vi "CheckPYME.vi"(0 "Anos de tu negocio":i32, 5 "Garantia":dbl, 7 "Importe total":dbl, 9 "Flujo de efectivo mensual":dbl, 11 "Numero de sucursales":i32) -> (6 "Sujeto a credito?":bool, 8 "Puntos momentaneos":i32, 10 "Status":string)   [LabVIEW 2018]
doc: "Verifica si la PYME esta sujeta a credito o no"
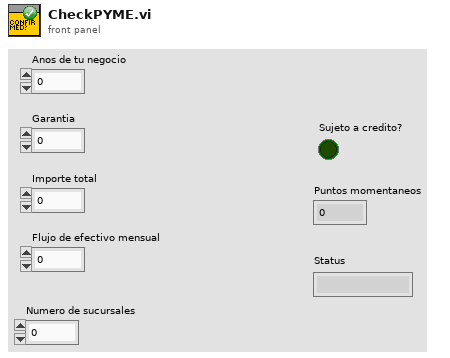
[diagram p1: front panel]
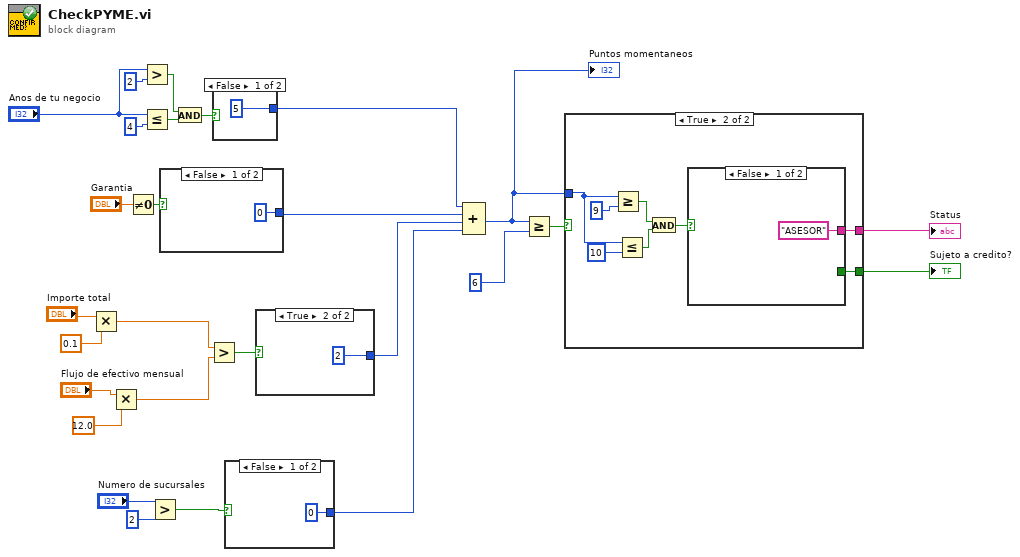
[diagram p0: block diagram]
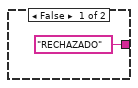
[diagram p2: hidden frame]
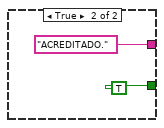
[diagram p3: hidden frame]
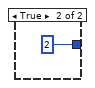
[diagram p4: hidden frame]
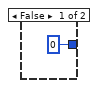
[diagram p5: hidden frame]
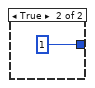
[diagram p6: hidden frame]
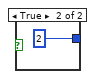
[diagram p7: hidden frame]
diagram:
  n1 = Multiply(x="Importe total", y=0.1) -> (x*y=w15:dbl)
  n2 = Multiply(x="Flujo de efectivo mensual", y=12.0) -> (x*y=w14:dbl)
  n3 = Not Equal To 0?(x="Garantia") -> (x != 0?=w20:bool)
  n4 = Greater?(x="Anos de tu negocio", y=2) -> (0:w24:bool)
  n5 = Less Or Equal?(x="Anos de tu negocio", y=4) -> (x <= y?=w23:bool)
  n6 = Greater?(x="Numero de sucursales", y=2) -> (0:w10:bool)
  n7 = case shown="False" w20 {
    tunnel: [0 1] -> w8
    frame False {
    }
    frame True {
    }
  }
  n8 = And(x=w24, y=w23) -> (x .and. y?=w22:bool)
  n9 = Greater?(x=w15, y=w14) -> (0:w13:bool)
  n10 = case shown="False" w22 {
    tunnel: [5 2] -> w9
    frame False {
    }
    frame True {
    }
  }
  n11 = case shown="False" w10 {
    tunnel: [0 2] -> w6
    frame False {
    }
    frame True {
    }
  }
  n12 = case shown="True" w13 {
    tunnel: [0 2] -> w7
    frame False {
    }
    frame True {
    }
  }
  n13 = Compound Arithmetic op=ADD(w9, w8, w7, w6) -> (w1:i32)
  "Puntos momentaneos" <- w1
  n14 = Greater Or Equal?(x=w1, y=6) -> (x >= y?=w4:bool)
  n15 = case shown="True" w4 {
    tunnel: w1 -> [_ w43]
    tunnel: ["RECHAZADO" ("Status") w38] -> w3
    tunnel: [_ w37] -> w2
    frame False {
    }
    frame True {
      n16 = Greater Or Equal?(x=w43, y=9) -> (x >= y?=w41:bool)
      n17 = Less Or Equal?(x=w43, y=10) -> (x <= y?=w40:bool)
      n18 = And(x=w41, y=w40) -> (x .and. y?=w39:bool)
      n19 = case shown="False" w39 {
        tunnel: ["ASESOR" ("Status") "ACREDITADO." ("Status")] -> w38
        tunnel: [_ TRUE ("Sujeto a credito?")] -> w37
        frame False {
        }
        frame True {
        }
      }
    }
  }
  "Sujeto a credito?" <- w2
  "Status" <- w3
